vi "_StopSignal-Signleton.vi"(0 "name(\"\")":string, 1 "Action":T2, 5 "StopSignal":T1, 7 "force destroy?(F)":bool, 11 "error in":errorcluster) -> (3 "AllSignalsInorder":string[](array[string]), 4 "StopSignalRef":T1, 6 "created new?":bool=TRUE, 8 "StopSignalLib":T3, 10 "name":string, 15 "error out":errorcluster)   [LabVIEW 2017, in "StopSignal.lvlib"]
uses:
  StopSignal.lvlib
  Typedef/Action.ctl
  Typedef/StopSignal.ctl
  API/StopSignal-IsValid.vi
  _Create.vi
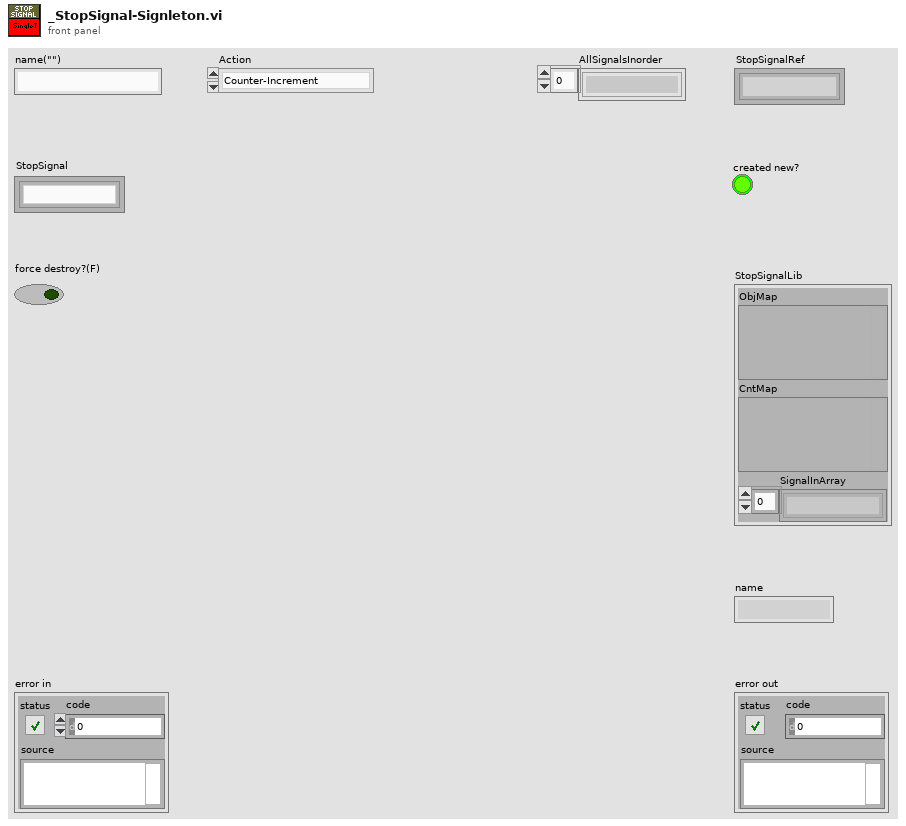
[diagram p1: front panel]
types:
  T1 = typedef "StopSignal.lvlib/StopSignal.ctl" = refnum<k1>
  T2 = typedef "StopSignal.lvlib/Action.ctl" = enum16{"Counter-Increment", "Counter-Decrement", "Counter-Name", "Get-All-Signals-Inorder", "Get-Stop-Signal-Lib"}
  T3 = cluster{"ObjMap":variant, "CntMap":variant, "SignalInArray":string[]}
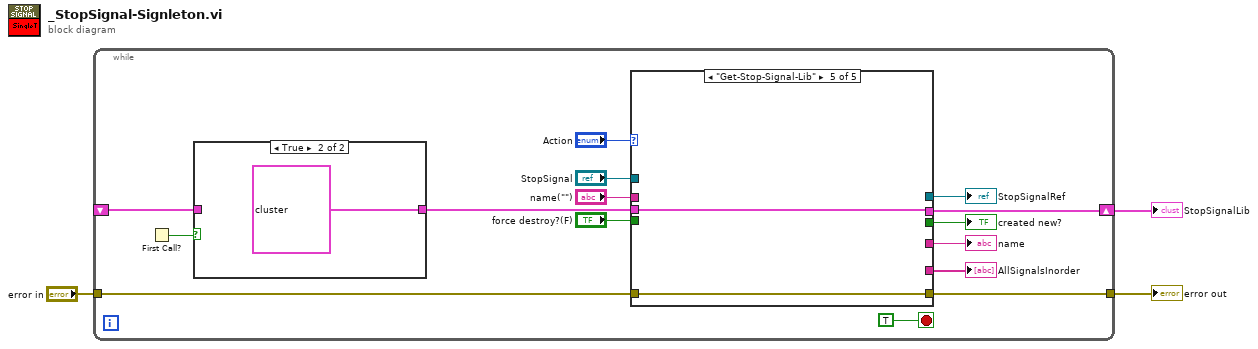
[diagram p0: block diagram]
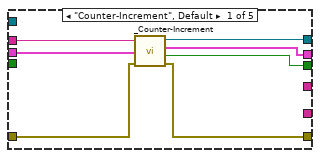
[diagram p3: hidden frame]
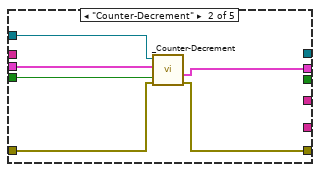
[diagram p4: hidden frame]
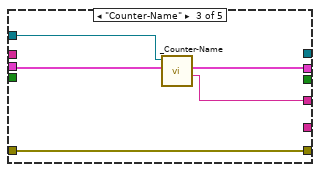
[diagram p5: hidden frame]
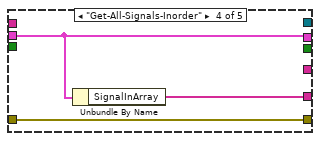
[diagram p6: hidden frame]
diagram:
  n1 = while {
    shift-right: [w17] -> w3
    shift-left: _ -> [w14]
    tunnel: "error in" -> [w9]
    tunnel: [w7] -> w1
    stop <- TRUE stop-if-true
    n2 = First Call?() -> (First Call?: T/F=w15:bool)
    n3 = case shown="True" w15 {
      tunnel: [w19 T3 {"ObjMap"=variant, "CntMap"=variant, "SignalInArray"=[]}] -> w13
      tunnel: w14 -> [w19 _]
      frame False {
      }
      frame True {
      }
    }
    n4 = case shown="\"Get-Stop-Signal-Lib\"" "Action" {
      tunnel: [w26 w32 w37 w40 w43] -> w17
      tunnel: w13 -> [w27 w33 w38 w40 w43]
      tunnel: "StopSignal" -> [_ w31 w36 _ _]
      tunnel: "force destroy?(F)" -> [_ w30 _ _ _]
      tunnel: "name(\"\")" -> [w25 _ _ _ _]
      tunnel: w9 -> [w24 w29 w35 w41 w42]
      tunnel: [w23 w28 w35 w41 w42] -> w7
      tunnel: [_ _ _ w39 _] -> w8
      tunnel: [w22 _ _ _ _] -> w6
      tunnel: [w21 _ _ _ _] -> w5
      tunnel: [_ _ w34 _ _] -> w4
      frame "Counter-Increment", Default {
        n5 = call "_Counter-Increment.vi"("error in"=w24, "StopSignalLib"=w27, "name(\"\")"=w25) -> ("error out"=w23:errorcluster, "created new?"=w21:bool, "cacher"=w26:T3, "StopSignalRef"=w22:T1)  [unwired: 5 in]
      }
      frame "Counter-Decrement" {
        n6 = call "_Counter-Decrement.vi"("error in (no error)"=w29, "force destroy?(F)"=w30, "StopSignalLib"=w33, "StopSignal"=w31) -> ("error out"=w28:errorcluster, "cache"=w32:T3)  [unwired: 6 in]
      }
      frame "Counter-Name" {
        n7 = call "_Counter-Name.vi"("StopSignalLib"=w38, "StopSignal"=w36) -> ("name"=w34:string, "StopSignalLib"=w37:T3)  [unwired: 7 in, 1 out]
      }
      frame "Get-All-Signals-Inorder" {
        n8 = Unbundle By Name(w40) -> ("SignalInArray"=w39:string[])
      }
      frame "Get-Stop-Signal-Lib" {
      }
    }
    "AllSignalsInorder" <- w8
    "StopSignalRef" <- w6
    "created new?" <- w5
    "name" <- w4
  }
  "StopSignalLib" <- w3
  "error out" <- w1
